vi "Manipulator PanelM.vi"() -> ()   [LabVIEW 2012]
uses:
  <vilib>/Platform/TimedLoop/XDataNode/timing_clust.ctl
  <vilib>/Platform/TimedLoop/XDataNode/nitl_modes.ctl
  <vilib>/Platform/TimedLoop/XDataNode/wakeup.ctl
  <vilib>/Utility/inputDevices.llb/joystickAcquire.vi
  <vilib>/Platform/TimedLoop/XDataNode/XDataNode.xnode
  <vilib>/Platform/TimedLoop/XDataNode/XDNodeRunTimeDep.lvlib
panel:
  in  "TCPConRef":refnum<k5>
  out "axis info":T1
  out "button info":T2
  in  "Joystick Selector":u16(ring) items=["Logitech Attack 3 USB", "USB Receiver", "USB Receiver", "USB Receiver", "USB Receiver", "USB Receiver", "USB Receiver"]
  in  "Use Joystick":bool
  out "Active":bool
  in  "Arm Rotate ccw":bool
  in  "Arm Rotate cw":bool
  in  "Claw close":bool
  in  "Claw open":bool
  in  "Arm right":bool
  in  "Arm left":bool
  in  "Lower arm down":bool
  in  "Lower arm up":bool
  in  "Upper arm down":bool
  in  "Upper arm up":bool
  in  "Power switch\nmanipulator":bool
  out "Reset":bool
  out "Turning off in":dbl=10.0
  # "JOYSTICK CONTROL"
  # "MANUAL CONTROL"
  # "INFO"
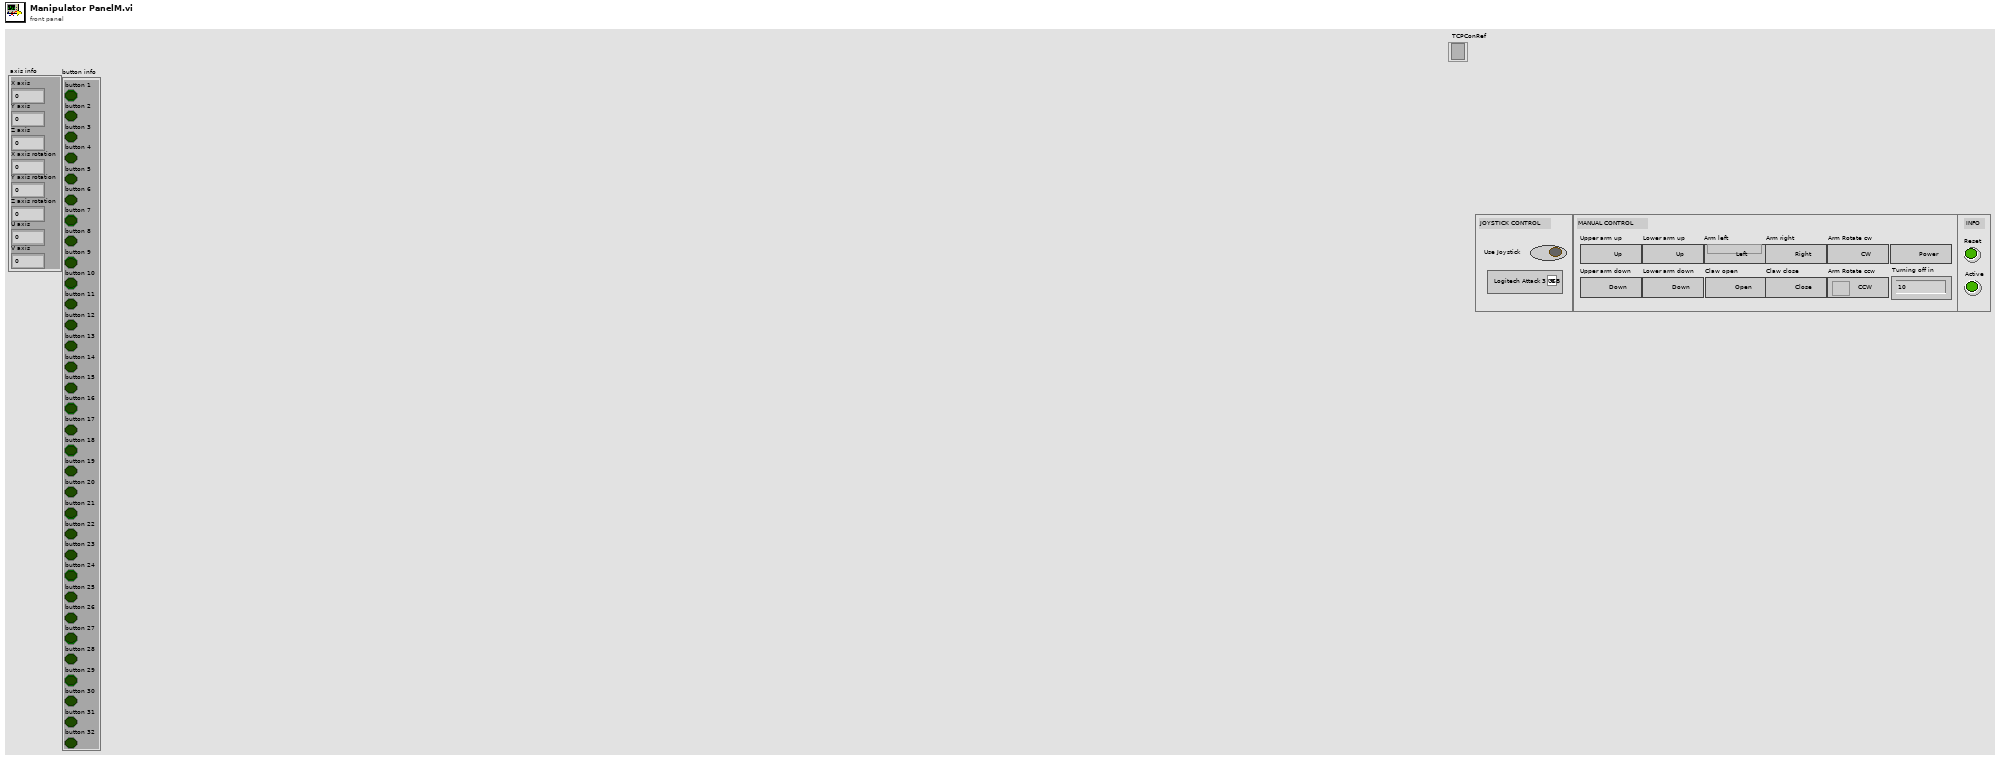
[diagram p1: front panel]
types:
  T1 = cluster{"X axis":i32, "Y axis":i32, "Z axis":i32, "X axis rotation":i32, "Y axis rotation":i32, "Z axis rotation":i32, "U axis":i32, "V axis":i32}
  T2 = cluster{"button 1":bool, "button 2":bool, "button 3":bool, "button 4":bool, "button 5":bool, "button 6":bool, "button 7":bool, "button 8":bool, "button 9":bool, "button 10":bool, "button 11":bool, "button 12":bool, "button 13":bool, "button 14":bool, "button 15":bool, "button 16":bool, "button 17":bool, "button 18":bool, "button 19":bool, "button 20":bool, "button 21":bool, "button 22":bool, "button 23":bool, "button 24":bool, "button 25":bool, "button 26":bool, "button 27":bool, "button 28":bool, "button 29":bool, "button 30":bool, "button 31":bool, "button 32":bool}
  T3 = typedef "XDNodeRunTimeDep.lvlib/timing_clust.ctl" = cluster{"Expected End [f-1]":u64, "Actual End [f-1]":u64, "Finished Late? [f-1]":bool, "Expected End [i-1]":u64, "Actual End [i-1]":u64, "Finished Late? [i-1]":bool, "Expected Start [i]":u64, "Actual Start [i]":u64, "Expected Start [f]":u64, "Actual Start [f]":u64, "Source Name":string, "Structure Name":string, "Period":i64, "Deadline":i64, "Offset":i64, "Start":i64, "Priority":i32, "Timeout":i32, "Mode":T4, "Wakeup Reason":T5, "Error":errorcluster, "Source Type":string, "Secondary Source Type":string, "Global End Time":u64, "Global Start Time":u64, "Frame Duration":u64, "Iteration Duration":u64, "Assigned CPU":i32, "I/O Scan Engine Mode":u32}
  T4 = typedef "XDNodeRunTimeDep.lvlib/nitl_modes.ctl" = enum32{"No Change", "Process missed periods, maintain original phase", "Discard missed periods, maintain original phase", "Process missed periods, ignore original phase", "Discard missed periods, ignore original phase"}
  T5 = typedef "XDNodeRunTimeDep.lvlib/wakeup.ctl" = enum32{"Normal", "Aborted", "Asynchronous wakeup", "Timing source error", "Timed loop error", "Timeout"}
  T6 = cluster{"axes total":u32, "buttons total":u32, "pov total":u32, "device name":string}[]
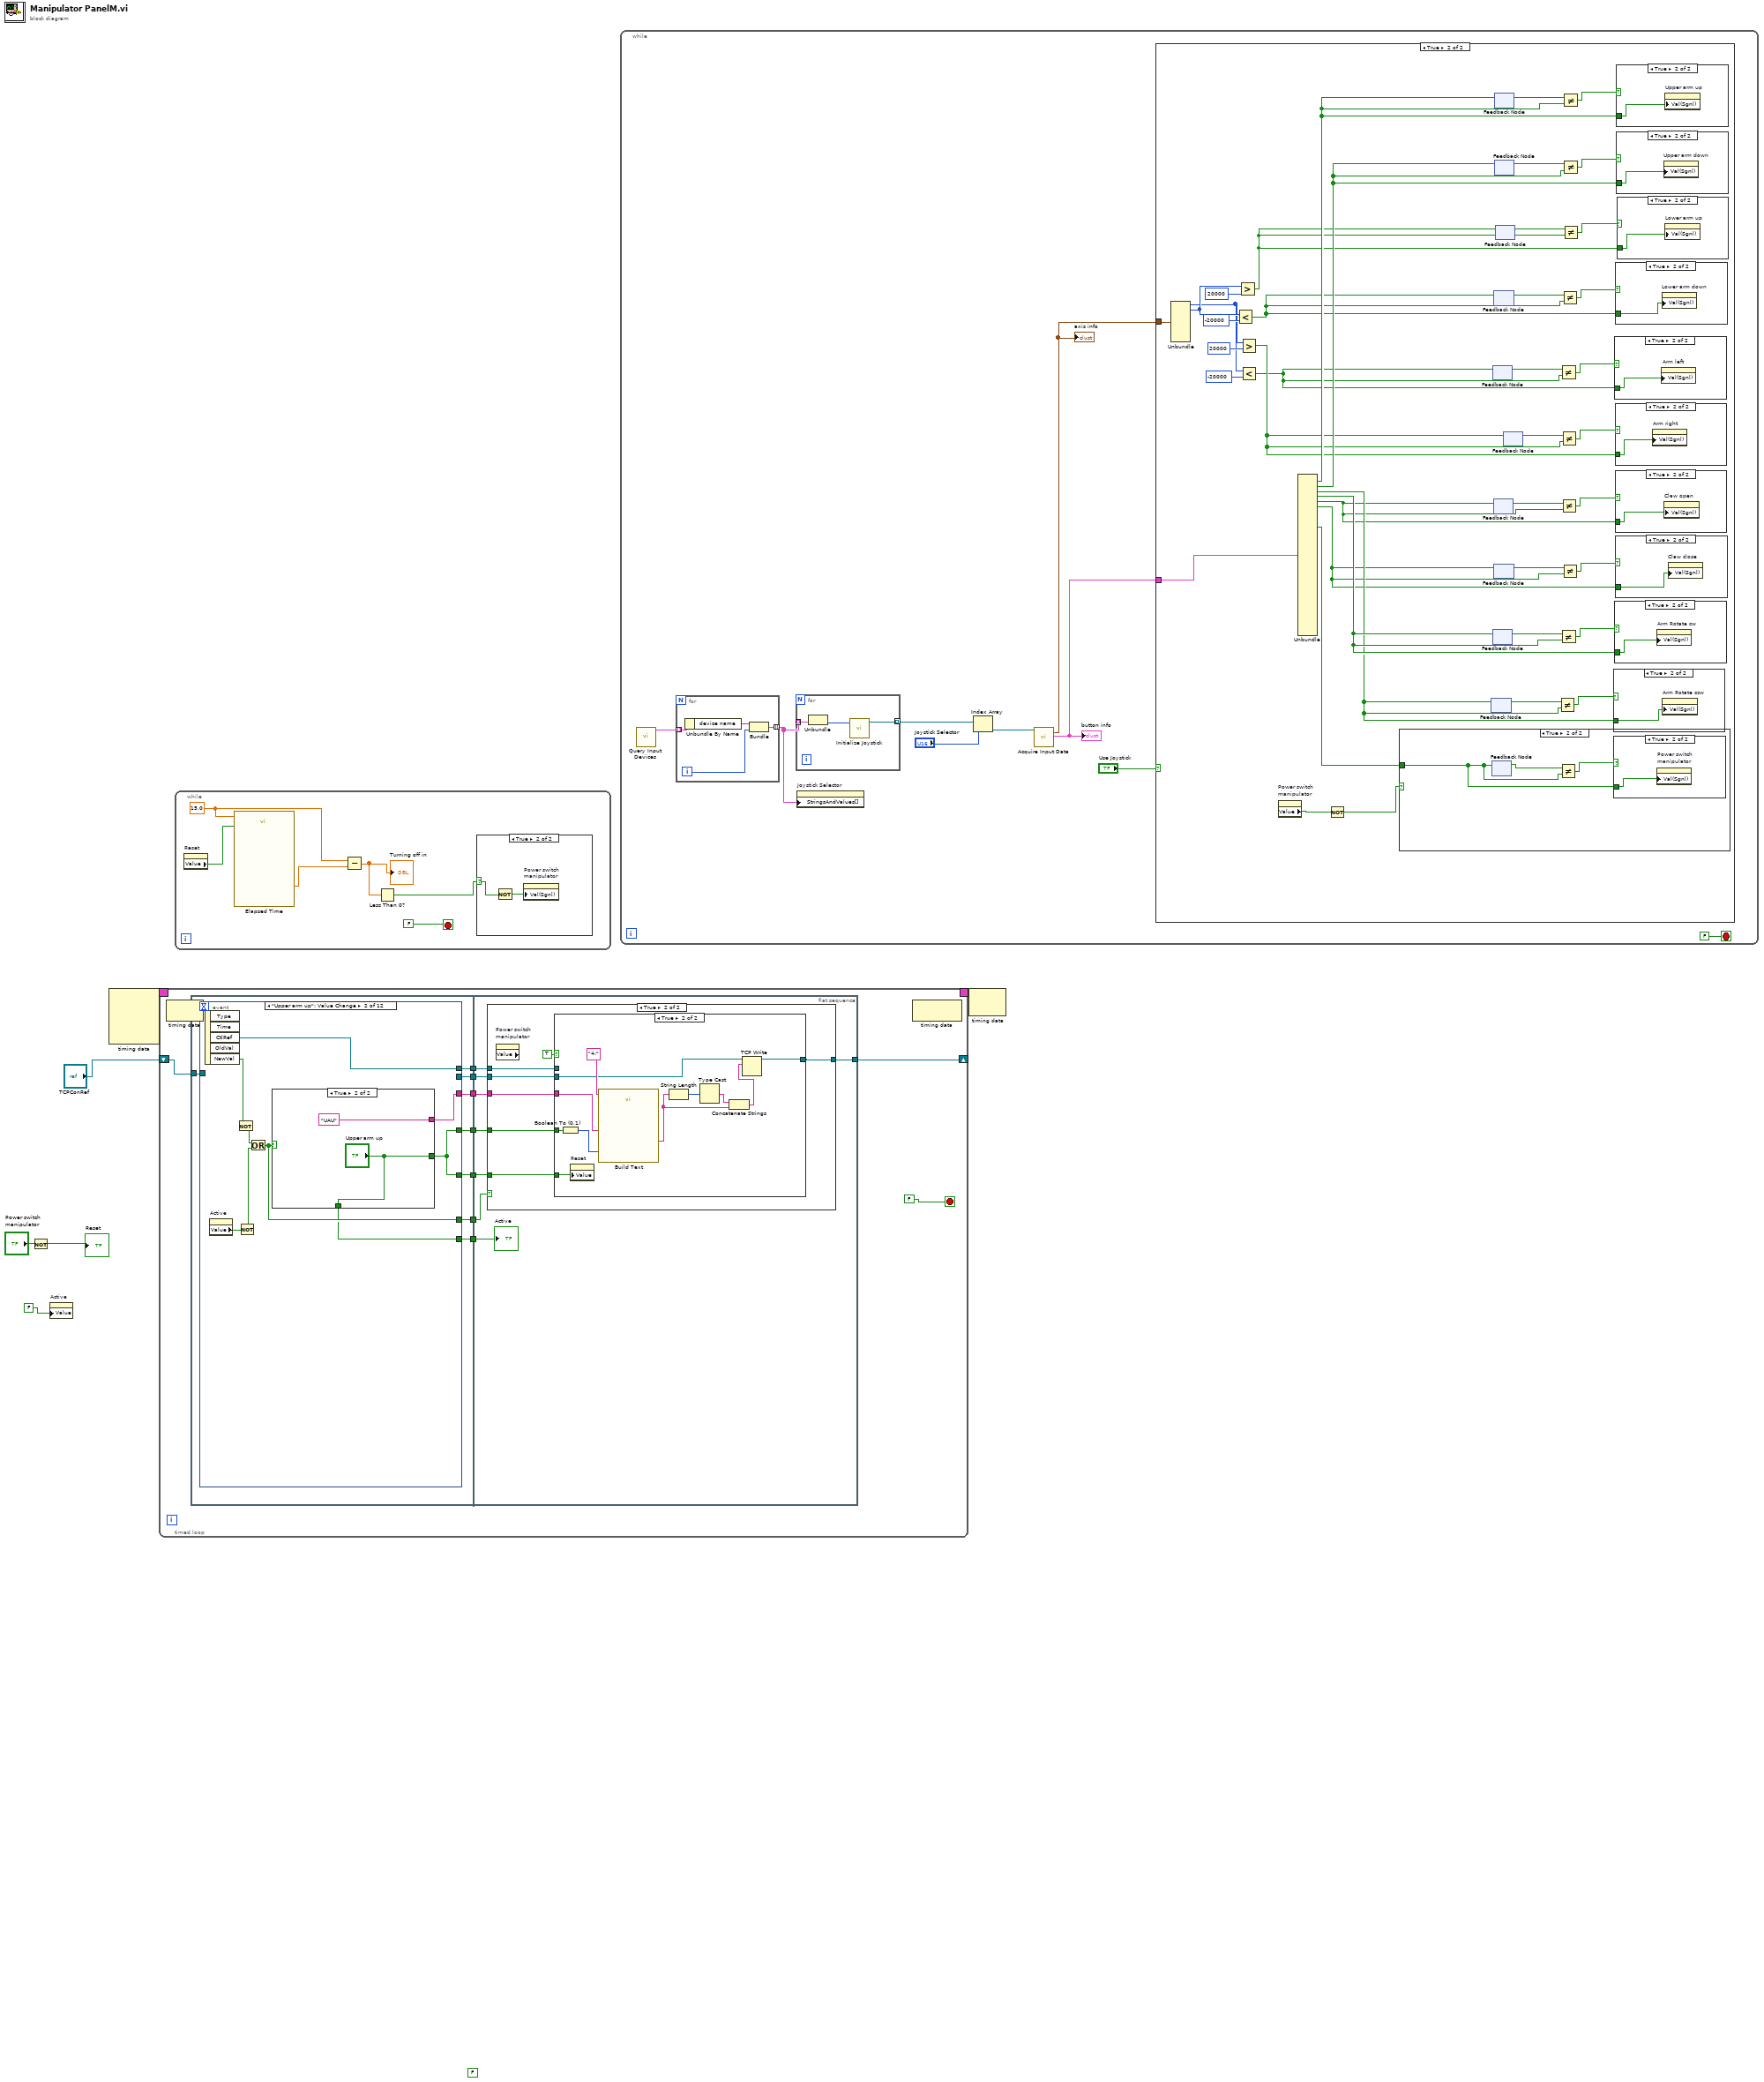
[diagram p0: block diagram]
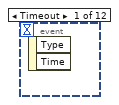
[diagram p15: hidden frame]
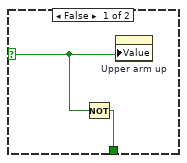
[diagram p16: hidden frame]
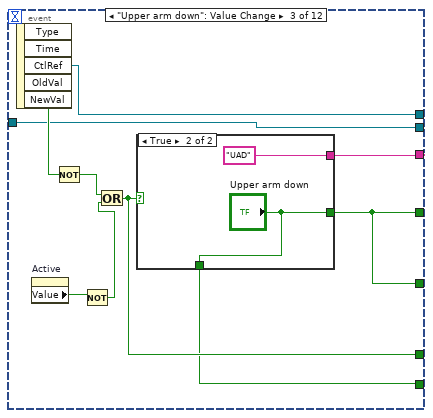
[diagram p17: hidden frame]
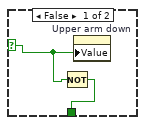
[diagram p18: hidden frame]
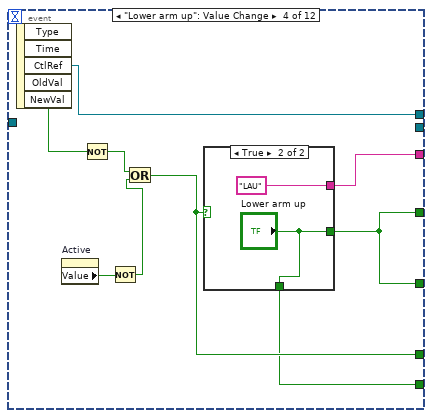
[diagram p19: hidden frame]
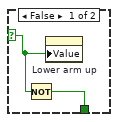
[diagram p20: hidden frame]
diagram:
  (unwired) FALSE
  n1 = Not(x="Power switch\nmanipulator") -> (.not. x?=→"Reset":bool)
  n2 = property on="Active" class="Bool (strict)"("Value"=FALSE) -> ()  [unwired: 2 in, 2 out]
  n3 = node-c288() -> (w6:T3)  [unwired: 4 in]
  n4 = timed-loop {
    timing: w6 -> [_]
    timing-out: [_] -> w5
    shift-right: [w9] -> _
    shift-left: "TCPConRef" -> [w7]
    stop <- FALSE stop-if-true
    n5 = node-c288() -> ()  [unwired: 1 in, 1 out]
    n6 = flat-sequence {
      tunnel: [w26] -> w15
      tunnel: [w25] -> w14
      tunnel: [w24] -> w13
      tunnel: [w23] -> w12
      tunnel: [w22] -> w11
      tunnel: [w21] -> w10
      tunnel: [w20] -> w8
      tunnel: w7 -> [w19]
      tunnel: w15 -> [w172]
      tunnel: w14 -> [w171]
      tunnel: w13 -> [w173]
      tunnel: w12 -> [w170]
      tunnel: w11 -> [w169]
      tunnel: w10 -> [w168]
      tunnel: [w167] -> w9
      tunnel: w8 -> [w166]
      frame #0 {
        n7 = event shown="[1] \"Upper arm up\": Value Change" {
          selector: _ -> [_ _ _ _ _ _ _ _ _ _ _ _]
          dyn-events: _ -> [_ _ _ _ _ _ _ _ _ _ _ _]
          timeout: _ -> [_ _ _ _ _ _ _ _ _ _ _ _]
          tunnel: [_ w30 w49 w61 w75 w88 w100 w114 w127 w139 w152 "PSM"] -> w26
          tunnel: [_ w29 w47 w62 w74 w87 w101 w112 w125 w140 w153 w162] -> w25
          tunnel: [_ w29 w47 w62 w74 w87 w101 w112 w125 w140 w153 w163] -> w23
          tunnel: [_ w35 w48 w60 w73 w86 w99 w113 w126 w138 w151 w161] -> w24
          tunnel: [_ w28 w42 w55 w68 w81 w94 w107 w120 w133 w146 w158] -> w22
          tunnel: [_ w27 w41 w54 w67 w80 w93 w106 w119 w132 w145 w159] -> w21
          tunnel: [_ _ w40 _ _ _ _ _ _ _ _ _] -> w20
          tunnel: w19 -> [_ _ w40 _ _ _ _ _ _ _ _ _]
          event Timeout {
            n8 = event-data() -> ()  [unwired: 1 in, 2 out]
          }
          event "Upper arm up": Value Change {
            n9 = event-data() -> ("CtlRef"=w35:refnum<vi>, "NewVal"=w34:bool)  [unwired: 1 in, 3 out]
            n10 = property on="Active" class="Bool (strict)"() -> ("Value"=w33:bool)  [unwired: 2 in, 2 out]
            n11 = Not(x=w34) -> (.not. x?=w31:bool)
            n12 = Not(x=w33) -> (.not. x?=w32:bool)
            n13 = Or(x=w31, y=w32) -> (x .or. y?=w28:bool)
            n14 = case shown="True" w28 {
              selector: w28 -> [w37 _]
              tunnel: [_ "UAU"] -> w30
              tunnel: [_ "Upper arm up"] -> w29
              tunnel: [w36 "Upper arm up"] -> w27
              frame False {
                n15 = Not(x=w37) -> (.not. x?=w36:bool)
                n16 = property on="Upper arm up" class="Bool (strict)"("Value"=w37) -> ()  [unwired: 2 in, 2 out]
              }
              frame True {
              }
            }
          }
          event "Upper arm down": Value Change {
            n17 = event-data() -> ("CtlRef"=w48:refnum<vi>, "NewVal"=w43:bool)  [unwired: 1 in, 3 out]
            n18 = property on="Active" class="Bool (strict)"() -> ("Value"=w46:bool)  [unwired: 2 in, 2 out]
            n19 = Not(x=w43) -> (.not. x?=w44:bool)
            n20 = Not(x=w46) -> (.not. x?=w45:bool)
            n21 = Or(x=w44, y=w45) -> (x .or. y?=w42:bool)
            n22 = case shown="True" w42 {
              selector: w42 -> [w51 _]
              tunnel: [_ "UAD"] -> w49
              tunnel: [_ "Upper arm down"] -> w47
              tunnel: [w50 "Upper arm down"] -> w41
              frame False {
                n23 = Not(x=w51) -> (.not. x?=w50:bool)
                n24 = property on="Upper arm down" class="Bool (strict)"("Value"=w51) -> ()  [unwired: 2 in, 2 out]
              }
              frame True {
              }
            }
          }
          event "Lower arm up": Value Change {
            n25 = event-data() -> ("CtlRef"=w60:refnum<vi>, "NewVal"=w59:bool)  [unwired: 1 in, 3 out]
            n26 = property on="Active" class="Bool (strict)"() -> ("Value"=w56:bool)  [unwired: 2 in, 2 out]
            n27 = Not(x=w59) -> (.not. x?=w58:bool)
            n28 = Not(x=w56) -> (.not. x?=w57:bool)
            n29 = Or(x=w58, y=w57) -> (x .or. y?=w55:bool)
            n30 = case shown="True" w55 {
              selector: w55 -> [w64 _]
              tunnel: [_ "Lower arm up"] -> w62
              tunnel: [_ "LAU"] -> w61
              tunnel: [w63 "Lower arm up"] -> w54
              frame False {
                n31 = Not(x=w64) -> (.not. x?=w63:bool)
                n32 = property on="Lower arm up" class="Bool (strict)"("Value"=w64) -> ()  [unwired: 2 in, 2 out]
              }
              frame True {
              }
            }
          }
          event "Lower arm down": Value Change {
            n33 = event-data() -> ("CtlRef"=w73:refnum<vi>, "NewVal"=w69:bool)  [unwired: 1 in, 3 out]
            n34 = property on="Active" class="Bool (strict)"() -> ("Value"=w72:bool)  [unwired: 2 in, 2 out]
            n35 = Not(x=w69) -> (.not. x?=w70:bool)
            n36 = Not(x=w72) -> (.not. x?=w71:bool)
            n37 = Or(x=w70, y=w71) -> (x .or. y?=w68:bool)
            n38 = case shown="False" w68 {
              selector: w68 -> [w76 _]
              tunnel: [_ "LAD"] -> w75
              tunnel: [_ "Lower arm down"] -> w74
              tunnel: [w77 "Lower arm down"] -> w67
              frame False {
                n39 = property on="Lower arm down" class="Bool (strict)"("Value"=w76) -> ()  [unwired: 2 in, 2 out]
                n40 = Not(x=w76) -> (.not. x?=w77:bool)
              }
              frame True {
              }
            }
          }
          event "Arm left": Value Change {
            n41 = event-data() -> ("CtlRef"=w86:refnum<vi>, "NewVal"=w84:bool)  [unwired: 1 in, 3 out]
            n42 = property on="Active" class="Bool (strict)"() -> ("Value"=w85:bool)  [unwired: 2 in, 2 out]
            n43 = Not(x=w84) -> (.not. x?=w83:bool)
            n44 = Not(x=w85) -> (.not. x?=w82:bool)
            n45 = Or(x=w83, y=w82) -> (x .or. y?=w81:bool)
            n46 = case shown="True" w81 {
              selector: w81 -> [w90 _]
              tunnel: [_ "MAL"] -> w88
              tunnel: [_ "Arm left"] -> w87
              tunnel: [w89 "Arm left"] -> w80
              frame False {
                n47 = Not(x=w90) -> (.not. x?=w89:bool)
                n48 = property on="Arm left" class="Bool (strict)"("Value"=w90) -> ()  [unwired: 2 in, 2 out]
              }
              frame True {
              }
            }
          }
          event "Arm right": Value Change {
            n49 = event-data() -> ("CtlRef"=w99:refnum<vi>, "NewVal"=w96:bool)  [unwired: 1 in, 3 out]
            n50 = property on="Active" class="Bool (strict)"() -> ("Value"=w95:bool)  [unwired: 2 in, 2 out]
            n51 = Not(x=w96) -> (.not. x?=w97:bool)
            n52 = Not(x=w95) -> (.not. x?=w98:bool)
            n53 = Or(x=w97, y=w98) -> (x .or. y?=w94:bool)
            n54 = case shown="True" w94 {
              selector: w94 -> [w103 _]
              tunnel: [_ "Arm right"] -> w101
              tunnel: [_ "MAR"] -> w100
              tunnel: [w102 "Arm right"] -> w93
              frame False {
                n55 = Not(x=w103) -> (.not. x?=w102:bool)
                n56 = property on="Arm right" class="Bool (strict)"("Value"=w103) -> ()  [unwired: 2 in, 2 out]
              }
              frame True {
              }
            }
          }
          event "Claw open": Value Change {
            n57 = event-data() -> ("CtlRef"=w113:refnum<vi>, "NewVal"=w111:bool)  [unwired: 1 in, 3 out]
            n58 = property on="Active" class="Bool (strict)"() -> ("Value"=w108:bool)  [unwired: 2 in, 2 out]
            n59 = Not(x=w111) -> (.not. x?=w110:bool)
            n60 = Not(x=w108) -> (.not. x?=w109:bool)
            n61 = Or(x=w110, y=w109) -> (x .or. y?=w107:bool)
            n62 = case shown="True" w107 {
              selector: w107 -> [w115 _]
              tunnel: [_ "CLO"] -> w114
              tunnel: [_ "Claw open"] -> w112
              tunnel: [w116 "Claw open"] -> w106
              frame False {
                n63 = Not(x=w115) -> (.not. x?=w116:bool)
                n64 = property on="Claw open" class="Bool (strict)"("Value"=w115) -> ()  [unwired: 2 in, 2 out]
              }
              frame True {
              }
            }
          }
          event "Claw close": Value Change {
            n65 = event-data() -> ("CtlRef"=w126:refnum<vi>, "NewVal"=w121:bool)  [unwired: 1 in, 3 out]
            n66 = property on="Active" class="Bool (strict)"() -> ("Value"=w122:bool)  [unwired: 2 in, 2 out]
            n67 = Not(x=w121) -> (.not. x?=w124:bool)
            n68 = Not(x=w122) -> (.not. x?=w123:bool)
            n69 = Or(x=w124, y=w123) -> (x .or. y?=w120:bool)
            n70 = case shown="True" w120 {
              selector: w120 -> [w129 _]
              tunnel: [_ "CLC"] -> w127
              tunnel: [_ "Claw close"] -> w125
              tunnel: [w128 "Claw close"] -> w119
              frame False {
                n71 = Not(x=w129) -> (.not. x?=w128:bool)
                n72 = property on="Claw close" class="Bool (strict)"("Value"=w129) -> ()  [unwired: 2 in, 2 out]
              }
              frame True {
              }
            }
          }
          event "Arm Rotate cw": Value Change {
            n73 = event-data() -> ("CtlRef"=w138:refnum<vi>, "NewVal"=w135:bool)  [unwired: 1 in, 3 out]
            n74 = property on="Active" class="Bool (strict)"() -> ("Value"=w134:bool)  [unwired: 2 in, 2 out]
            n75 = Not(x=w135) -> (.not. x?=w136:bool)
            n76 = Not(x=w134) -> (.not. x?=w137:bool)
            n77 = Or(x=w136, y=w137) -> (x .or. y?=w133:bool)
            n78 = case shown="True" w133 {
              selector: w133 -> [w142 _]
              tunnel: [_ "Arm Rotate cw"] -> w140
              tunnel: [_ "ARR"] -> w139
              tunnel: [w141 "Arm Rotate cw"] -> w132
              frame False {
                n79 = Not(x=w142) -> (.not. x?=w141:bool)
                n80 = property on="Arm Rotate cw" class="Bool (strict)"("Value"=w142) -> ()  [unwired: 2 in, 2 out]
              }
              frame True {
              }
            }
          }
          event "Arm Rotate ccw": Value Change {
            n81 = event-data() -> ("CtlRef"=w151:refnum<vi>, "NewVal"=w148:bool)  [unwired: 1 in, 3 out]
            n82 = property on="Active" class="Bool (strict)"() -> ("Value"=w147:bool)  [unwired: 2 in, 2 out]
            n83 = Not(x=w148) -> (.not. x?=w149:bool)
            n84 = Not(x=w147) -> (.not. x?=w150:bool)
            n85 = Or(x=w149, y=w150) -> (x .or. y?=w146:bool)
            n86 = case shown="True" w146 {
              selector: w146 -> [w155 _]
              tunnel: [_ "Arm Rotate ccw"] -> w153
              tunnel: [_ "ARL"] -> w152
              tunnel: [w154 "Arm Rotate ccw"] -> w145
              frame False {
                n87 = Not(x=w155) -> (.not. x?=w154:bool)
                n88 = property on="Arm Rotate ccw" class="Bool (strict)"("Value"=w155) -> ()  [unwired: 2 in, 2 out]
              }
              frame True {
              }
            }
          }
          event "Power switch\nmanipulator": Value Change {
            w158 = TRUE
            n89 = event-data() -> ("CtlRef"=w161:refnum<vi>, "NewVal"=w160:bool)  [unwired: 1 in, 3 out]
            n90 = case shown="False" w160 {
              frame False {
                w165 = FALSE
                n91 = property on="Lower arm down" class="Bool (strict)"("Value"=w165) -> ()  [unwired: 2 in, 2 out]
                n92 = property on="Arm left" class="Bool (strict)"("Value"=w165) -> ()  [unwired: 2 in, 2 out]
                n93 = property on="Lower arm up" class="Bool (strict)"("Value"=w165) -> ()  [unwired: 2 in, 2 out]
                n94 = property on="Upper arm down" class="Bool (strict)"("Value"=w165) -> ()  [unwired: 2 in, 2 out]
                n95 = property on="Arm right" class="Bool (strict)"("Value"=w165) -> ()  [unwired: 2 in, 2 out]
                n96 = property on="Upper arm up" class="Bool (strict)"("Value"=w165) -> ()  [unwired: 2 in, 2 out]
                n97 = property on="Claw open" class="Bool (strict)"("Value"=w165) -> ()  [unwired: 2 in, 2 out]
                n98 = property on="Claw close" class="Bool (strict)"("Value"=w165) -> ()  [unwired: 2 in, 2 out]
                n99 = property on="Arm Rotate cw" class="Bool (strict)"("Value"=w165) -> ()  [unwired: 2 in, 2 out]
                n100 = property on="Arm Rotate ccw" class="Bool (strict)"("Value"=w165) -> ()  [unwired: 2 in, 2 out]
              }
              frame True {
              }
            }
            n101 = property on="Power switch\nmanipulator" class="Bool (strict)"() -> ("Value"=w162:bool)  [unwired: 2 in, 2 out]
            n102 = Not(x=w162) -> (.not. x?=w163:bool)
            n103 = Not(x=w158) -> (.not. x?=w159:bool)
          }
        }
      }
      frame #1 {
        n104 = case shown="True" w169 {
          tunnel: w173 -> [_ w181]
          tunnel: w172 -> [_ w180]
          tunnel: w171 -> [_ w179]
          tunnel: w170 -> [_ w178]
          tunnel: [w174 w176] -> w167
          tunnel: w166 -> [w174 w175]
          frame False {
          }
          frame True {
            n105 = property on="Power switch\nmanipulator" class="Bool (strict)" props=["Value"]() -> ()  [unwired: 2 in, 3 out]
            n106 = case shown="True" TRUE {
              tunnel: w180 -> [_ w202]
              tunnel: w179 -> [_ w197]
              tunnel: w181 -> [w184 _]
              tunnel: w178 -> [_ w195]
              tunnel: [w182 w194] -> w176
              tunnel: w175 -> [w182 w193]
              frame False {
                n107 = control-ref of="Power switch\nmanipulator"() -> (w185:refnum<vi>)
                n108 = Not Equal?(x=w184, y=w185) -> (x != y?=w183:bool)
                n109 = case shown="True" w183 {
                  tunnel: w184 -> [w188 w190]
                  frame False {
                    n110 = property class="Bool (strict)"(reference=w188) -> ("Value"=w187:bool)  [unwired: 1 in, 2 out]
                    n111 = Not(x=w187) -> (.not. x?=w186:bool)
                    n112 = property on="Reset" class="Bool (strict)"("Value"=w186) -> ()  [unwired: 2 in, 2 out]
                  }
                  frame True {
                    n113 = property class="Bool (strict)"(reference=w190, "Value"=FALSE) -> ()  [unwired: 1 in, 2 out]
                    n114 = One Button Dialog(message="You must start the\nmanipulator engine first") -> ()  [unwired: 1 in, 1 out]
                  }
                }
              }
              frame True {
                n115 = Boolean To (0,1)(Boolean=w197) -> (0, 1=w196:i16)
                n116 = property on="Reset" class="Bool (strict)"("Value"=w195) -> ()  [unwired: 2 in, 2 out]
                n117 = call "Build Text"("Beginning Text"="4:", "ControlID"=w202, "Bool"=w196) -> ("Result"=w198:string)  [unwired: 11 in, 1 out]
                n118 = String Length(string=w198) -> (length=w200:i32)
                n119 = Type Cast(x=w200) -> (*(type *) &x=w199:string)  [unwired: 1 in]
                n120 = Concatenate Strings(w199, w198) -> (w192:string)
                n121 = TCP Write(connection ID=w193, data in=w192) -> (connection ID out=w194:refnum<k5>)  [unwired: 2 in, 2 out]
              }
            }
          }
        }
        "Active" <- w168
      }
    }
    n122 = node-c288() -> ()  [unwired: 1 in, 1 out]
  }
  n123 = while {
    stop <- FALSE stop-if-true
    w208 = 15.0
    n124 = property on="Reset" class="Bool (strict)"() -> ("Value"=w205:bool)  [unwired: 2 in, 2 out]
    n125 = call "Elapsed Time"("Time Target (s)"=w208, "Reset"=w205) -> ("Elapsed Time (s)"=w207:dbl)  [unwired: 10 in, 7 out]
    n126 = Subtract(x=w208, y=w207) -> (x-y=w204:dbl)
    "Turning off in" <- w204
    n127 = Less Than 0?(x=w204) -> (x < 0?=w203:bool)
    n128 = case shown="True" w203 {
      selector: w203 -> [_ w209]
      frame False {
      }
      frame True {
        n129 = Not(x=w209) -> (.not. x?=w210:bool)
        n130 = property on="Power switch\nmanipulator" class="Bool (strict)"("Val(Sgnl)"=w210) -> ()  [unwired: 2 in, 2 out]
      }
    }
  }
  n131 = while {
    stop <- FALSE stop-if-true
    n132 = call <vilib>:"Query Input Devices.vi"() -> ("joystick info"=w217:T6)  [unwired: 8 in, 3 out]
    n133 = for {
      tunnel: w217 -> [w278] mode=indexing
      tunnel: [w275] -> w218 mode=indexing
      i -> [w276]
      n134 = Unbundle By Name(w278) -> ("device name"=w277:string)
      n135 = Bundle("device name"=w277, w276) -> (w275:cluster{"device name":string, i32})  [unwired: 1 in]
    }
    n136 = for {
      tunnel: w218 -> [w280] mode=indexing
      tunnel: [w281] -> w219 mode=indexing
      n137 = Unbundle(w280) -> (w279:i32)  [unwired: 1 out]
      n138 = call <vilib>:"Initialize Joystick.vi"("device index"=w279) -> ("device ID"=w281:refnum<k1>)  [unwired: 9 in, 1 out]
    }
    n139 = property on="Joystick Selector" class="Ring (strict)"("StringsAndValues[]"=w218) -> ()  [unwired: 2 in, 2 out]
    n140 = Index Array(array=w219, index="Joystick Selector") -> (element=w215:refnum<k1>)
    n141 = call-poly <vilib>:"Acquire Input Data.vi"("device ID"=w215) -> ("axis info"=w211:T1, "button info"=w213:T2)  [unwired: 14 in, 3 out]
    "axis info" <- w211
    "button info" <- w213
    n142 = case shown="True" "Use Joystick" {
      tunnel: w213 -> [_ w260]
      tunnel: w211 -> [_ w233]
      frame False {
      }
      frame True {
        n143 = Unbundle(w233) -> ("X axis"=w225:i32, "Y axis"=w230:i32)  [unwired: 6 out]
        n144 = Less?(x=w230, y=-20000) -> (x < y?=w231:bool)
        n145 = Greater?(x=w230, y=20000) -> (0:w228:bool)
        n146 = Greater?(x=w225, y=20000) -> (0:w224:bool)
        n147 = Less?(x=w225, y=-20000) -> (x < y?=w223:bool)
        n148 = property on="Power switch\nmanipulator" class="Bool (strict)"() -> ("Value"=w221:bool)  [unwired: 2 in, 2 out]
        n149 = Unbundle(w260) -> ("button 2"=w238:bool, "button 3"=w239:bool, "button 4"=w236:bool, "button 5"=w237:bool, "button 6"=w235:bool, "button 7"=w234:bool, "button 11"=w222:bool)  [unwired: 25 out]
        n150 = Not(x=w221) -> (.not. x?=w220:bool)
        n151 = case shown="True" w220 {
          tunnel: w222 -> [_ w261]
          frame False {
          }
          frame True {
            n152 = feedback #1() -> (w263:bool)  [unwired: 1 in]
            n153 = feedback-in #1(w261) -> ()
            n154 = Not Equal?(x=w263, y=w261) -> (x != y?=w262:bool)
            n155 = case shown="True" w262 {
              tunnel: w261 -> [_ w264]
              frame False {
              }
              frame True {
                n156 = property on="Power switch\nmanipulator" class="Bool (strict)"("Val(Sgnl)"=w264) -> ()  [unwired: 2 in, 2 out]
              }
            }
          }
        }
        n157 = feedback #2() -> (w252:bool)  [unwired: 1 in]
        n158 = feedback-in #2(w236) -> ()
        n159 = feedback #3() -> (w249:bool)  [unwired: 1 in]
        n160 = feedback-in #3(w223) -> ()
        n161 = feedback #4() -> (w255:bool)  [unwired: 1 in]
        n162 = feedback-in #4(w237) -> ()
        n163 = feedback-in #5(w235) -> ()
        n164 = feedback #5() -> (w259:bool)  [unwired: 1 in]
        n165 = feedback #6() -> (w246:bool)  [unwired: 1 in]
        n166 = feedback-in #6(w231) -> ()
        n167 = feedback #7() -> (w256:bool)  [unwired: 1 in]
        n168 = feedback-in #7(w234) -> ()
        n169 = feedback #8() -> (w241:bool)  [unwired: 1 in]
        n170 = feedback-in #8(w238) -> ()
        n171 = feedback #9() -> (w242:bool)  [unwired: 1 in]
        n172 = feedback-in #9(w239) -> ()
        n173 = feedback #10() -> (w245:bool)  [unwired: 1 in]
        n174 = feedback-in #10(w228) -> ()
        n175 = feedback #11() -> (w250:bool)  [unwired: 1 in]
        n176 = feedback-in #11(w224) -> ()
        n177 = Not Equal?(x=w252, y=w236) -> (x != y?=w253:bool)
        n178 = Not Equal?(x=w249, y=w223) -> (x != y?=w248:bool)
        n179 = Not Equal?(x=w255, y=w237) -> (x != y?=w254:bool)
        n180 = Not Equal?(x=w250, y=w224) -> (x != y?=w251:bool)
        n181 = Not Equal?(x=w259, y=w235) -> (x != y?=w258:bool)
        n182 = Not Equal?(x=w246, y=w231) -> (x != y?=w247:bool)
        n183 = Not Equal?(x=w256, y=w234) -> (x != y?=w257:bool)
        n184 = Not Equal?(x=w241, y=w238) -> (x != y?=w240:bool)
        n185 = Not Equal?(x=w242, y=w239) -> (x != y?=w243:bool)
        n186 = Not Equal?(x=w245, y=w228) -> (x != y?=w244:bool)
        n187 = case shown="True" w253 {
          tunnel: w236 -> [_ w271]
          frame False {
          }
          frame True {
            n188 = property on="Arm Rotate ccw" class="Bool (strict)"("Val(Sgnl)"=w271) -> ()  [unwired: 2 in, 2 out]
          }
        }
        n189 = case shown="True" w248 {
          tunnel: w223 -> [_ w267]
          frame False {
          }
          frame True {
            n190 = property on="Arm left" class="Bool (strict)"("Val(Sgnl)"=w267) -> ()  [unwired: 2 in, 2 out]
          }
        }
        n191 = case shown="True" w254 {
          tunnel: w237 -> [_ w272]
          frame False {
          }
          frame True {
            n192 = property on="Arm Rotate cw" class="Bool (strict)"("Val(Sgnl)"=w272) -> ()  [unwired: 2 in, 2 out]
          }
        }
        n193 = case shown="True" w251 {
          tunnel: w224 -> [_ w266]
          frame False {
          }
          frame True {
            n194 = property on="Arm right" class="Bool (strict)"("Val(Sgnl)"=w266) -> ()  [unwired: 2 in, 2 out]
          }
        }
        n195 = case shown="True" w258 {
          tunnel: w235 -> [_ w274]
          frame False {
          }
          frame True {
            n196 = property on="Claw open" class="Bool (strict)"("Val(Sgnl)"=w274) -> ()  [unwired: 2 in, 2 out]
          }
        }
        n197 = case shown="True" w247 {
          tunnel: w231 -> [_ w268]
          frame False {
          }
          frame True {
            n198 = property on="Lower arm down" class="Bool (strict)"("Val(Sgnl)"=w268) -> ()  [unwired: 2 in, 2 out]
          }
        }
        n199 = case shown="True" w257 {
          tunnel: w234 -> [_ w273]
          frame False {
          }
          frame True {
            n200 = property on="Claw close" class="Bool (strict)"("Val(Sgnl)"=w273) -> ()  [unwired: 2 in, 2 out]
          }
        }
        n201 = case shown="True" w240 {
          tunnel: w238 -> [_ w265]
          frame False {
          }
          frame True {
            n202 = property on="Upper arm up" class="Bool (strict)"("Val(Sgnl)"=w265) -> ()  [unwired: 2 in, 2 out]
          }
        }
        n203 = case shown="True" w243 {
          tunnel: w239 -> [_ w270]
          frame False {
          }
          frame True {
            n204 = property on="Upper arm down" class="Bool (strict)"("Val(Sgnl)"=w270) -> ()  [unwired: 2 in, 2 out]
          }
        }
        n205 = case shown="True" w244 {
          tunnel: w228 -> [_ w269]
          frame False {
          }
          frame True {
            n206 = property on="Lower arm up" class="Bool (strict)"("Val(Sgnl)"=w269) -> ()  [unwired: 2 in, 2 out]
          }
        }
      }
    }
  }
  n207 = node-c288(w5) -> ()  [unwired: 1 out]
